vi "init_AH2700.vi"   [LabVIEW 2019]
uses:
  Global/Global Variables/global.vi
  Global/Global Variables/Data_Display_global.vi
types:
  T1 = typedef "AH2700-Cluster.ctl" = cluster{"Units Display":i32, "Sample Switch":i32, "Frequency":dbl, "V excitation":dbl, "Capacity Graphic":dbl[][], "Loss Graphic":dbl[][], "Capacity":dbl, "Loss":dbl, "Update AH2500":bool, "Bias ":dbl, " AVerage":dbl}
  T2 = typedef "AH2700-Control.ctl" = cluster{"Update AH2500":bool}
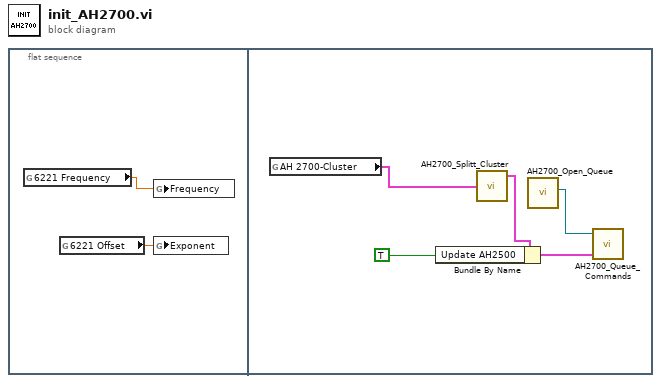
[diagram p0: block diagram]
diagram:
  n1 = flat-sequence {
    frame #0 {
      n2 = global read "global.vi" "6221 Frequency"() -> (w2:dbl)
      n3 = global read "global.vi" "6221 Offset"() -> (w1:dbl)
      n4 = global write "global.vi" "Frequency"(w2) -> ()
      n5 = global write "global.vi" "Exponent"(w1) -> ()
    }
    frame #1 {
      n6 = global read "Data_Display_global.vi" "AH 2700-Cluster"() -> (w7:T1)
      n7 = call "AH2700_Splitt_Cluster.vi"("AH 2700-Cluster"=w7) -> ("AH2700-Control"=w6:T2)  [unwired: 1 in, 1 out]
      n8 = Bundle By Name(cluster=w6, "Update AH2500"=TRUE) -> (w3:T2)
      n9 = call "AH2700_Open_Queue.vi"() -> ("queue out"=w4:refnum<queue>)  [unwired: 10 in, 1 out]
      n10 = call "AH2700_Queue_Commands.vi"("AH2700-Control"=w3, "AH2700 Queue"=w4) -> ()  [unwired: 1 in, 1 out]
    }
  }
